vi "Read Eulogy Bookmarks.vi"(8 "Error In":errorcluster, 11 "State In":T1) -> (0 "Error Out":errorcluster, 3 "State Out":T1)   [LabVIEW 2017, in "Bookmark Manager.lvlib"]
uses:
  Bookmark Manager.lvlib
  State.ctl
  VI Bookmark.ctl
  VI Information.ctl
  Application Information.ctl
  Bookmarks Views.ctl
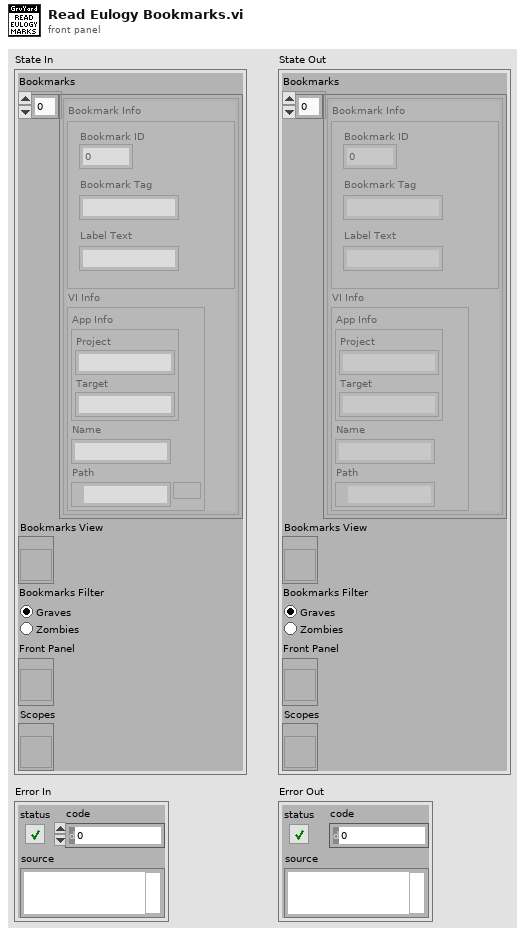
[diagram p1: front panel]
types:
  T1 = typedef "Bookmark Manager.lvlib/State.ctl" = cluster{"Bookmarks":T2[], "Bookmarks View":refnum<vi>, "Bookmarks Filter":T5, "Front Panel":refnum<vi>, "Scopes":refnum<vi>}
  T2 = typedef "Bookmark Manager.lvlib/VI Bookmark.ctl" = cluster{"Bookmark Info":cluster{"Bookmark ID":u32, "Bookmark Tag":string, "Label Text":string}, "VI Info":T3}
  T3 = typedef "Bookmark Manager.lvlib/VI Information.ctl" = cluster{"App Info":T4, "Name":string, "Path":path}
  T4 = typedef "Bookmark Manager.lvlib/Application Information.ctl" = cluster{"Project":string, "Target":string}
  T5 = typedef "Bookmark Manager.lvlib/Bookmarks Views.ctl" = enum32{"Graves", "Zombies"}
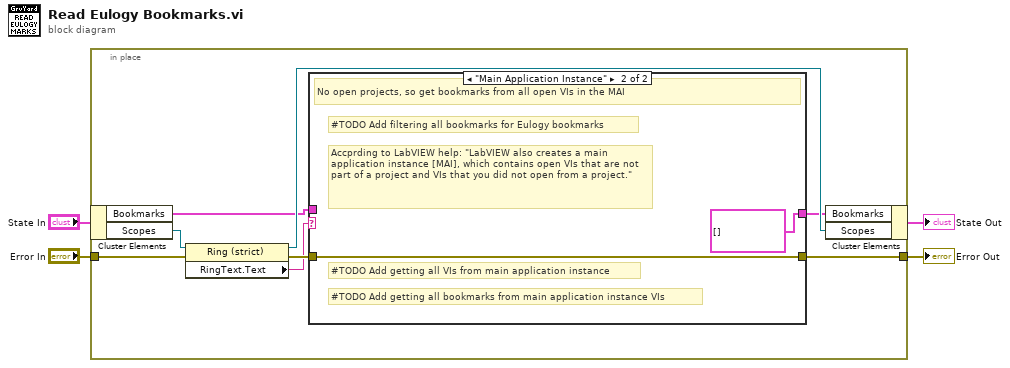
[diagram p0: block diagram]
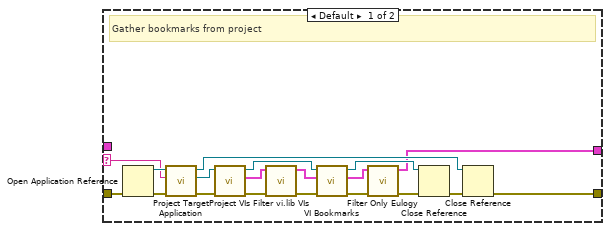
[diagram p2: hidden frame]
diagram:
  n1 = in-place {
    in-place-border: "Error In" -> [w12]
    in-place-border: [w11] -> w2
    n2 = in-place-cluster #1("State In") -> ("Bookmarks"=w5:T2[], "Scopes"=w9:refnum<vi>)
    n3 = property class="Ring (strict)"(reference=w9, error in=w12) -> (reference out=w7:refnum<vi>, error out=w10:errorcluster, "RingText.Text"=w8:string)
    n4 = case shown="\"Main Application Instance\"" w8 {
      selector: w8 -> [w28 _]
      tunnel: w10 -> [w31 w33]
      tunnel: [w27 w33] -> w11
      tunnel: [w13 T2[] [] ("Eulogy Bookmarks")] -> w6
      tunnel: w5 -> [_ _]
      frame Default {
        # "Gather bookmarks from project"
        n5 = Open Application Reference(8:w31) -> (0:w29:errorcluster, 3:w30:refnum<vi>)  [unwired: 3 in]
        n6 = call "Project Target Application.vi"("Error In"=w29, "Project Name"=w28, "App In"=w30) -> ("Error Out"=w25:errorcluster, "Project Target App"=w24:refnum<vi>, "App Out"=w26:refnum<vi>)  [unwired: 6 in]
        n7 = call "Project VIs.vi"("Error In"=w25, "Proejct Target App In"=w24) -> ("Error Out"=w21:errorcluster, "VIs"=w22:T3[], "Project Target App Out"=w18:refnum<vi>)  [unwired: 7 in]
        n8 = call "Filter vi.lib VIs.vi"("Error In"=w21, "VIs In"=w22) -> ("Error Out"=w20:errorcluster, "VIs Out"=w19:T3[])  [unwired: 8 in]
        n9 = call "VI Bookmarks.vi"("Error In"=w20, "VIs"=w19, "Project Target App In"=w18) -> ("Error Out"=w16:errorcluster, "VI Bookmarks"=w14:T2[], "Project Target App Out"=w17:refnum<vi>)  [unwired: 6 in]
        n10 = call "Filter Only Eulogy.vi"("Error In"=w16, "VI Bookmarks"=w14) -> ("Error Out"=w15:errorcluster, "Eulogy Bookmarks"=w13:T2[])  [unwired: 8 in]
        n11 = Close Reference(reference=w17, error in (no error)=w15) -> (error out=w23:errorcluster)
        n12 = Close Reference(reference=w26, error in (no error)=w23) -> (error out=w27:errorcluster)
      }
      frame "Main Application Instance" {
        # "#TODO Add filtering all bookmarks for Eulogy bookmarks"
        # "#TODO Add getting all bookmarks from main application instance VIs"
        # "#TODO Add getting all VIs from main application instance"
        # "Accprding to LabVIEW help: \"LabVIEW also creates a main application instance [MAI], which contains open VIs that are not part of a project and VIs that you did not open from a project.\""
        # "No open projects, so get bookmarks from all open VIs in the MAI"
      }
    }
    n13 = in-place-cluster #1("Bookmarks"=w6, "Scopes"=w7) -> (→"State Out":T1)
  }
  "Error Out" <- w2
